vi "Auton Reaquire.vi"   [LabVIEW 2015]
uses:
  Robot Values.vi
types:
  T1 = typedef "Robot Values.ctl" = cluster{"Drive Motors":cluster{"Left Motor Value":dbl, "Right Motor Value":dbl, "Left Motor Encoder":dbl, "Right Motor Encoder":dbl, "High/Low Gear":bool}, "Sensors":cluster{"Gyro Angle":dbl, "Photoeye":bool, "Ultrasonic Range":dbl, "Shooter Speed Encoder":dbl, "Accelerometer Value":dbl, "Flashlight":bool, "Target Distance":dbl, "Target X Value":dbl, "Reset Gyro?":bool}, "Arms":cluster{"Desired Arm Position":dbl, "Left Arm Encoder":dbl, "Right Arm Encoder":dbl, "Left Arm Lower Limit":bool, "Right Arm Lower Limit":bool, "Initialize Arm Position?":bool}, "Acquisition and Scoring":cluster{"Acquiring?":bool, "Current Speed":dbl, "Setpoint Speed":dbl, "Prep Wheels":bool, "Shoot":bool, "Low Eject":bool, "Reverse Shooter Wheel":bool}, "Hanging":cluster{"Pivot Arms":dbl, "PTO":bool, "Left Pivot Encoder":dbl, "Right Pivot Encoder":dbl, "Hanging Pin":bool}}
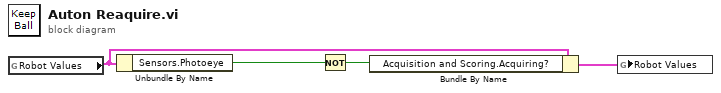
[diagram p0: block diagram]
diagram:
  n1 = global read "Robot Values.vi" "Robot Values"() -> (w4:T1)
  n2 = Unbundle By Name(w4) -> ("Sensors.Photoeye"=w3:bool)
  n3 = Not(x=w3) -> (.not. x?=w2:bool)
  n4 = Bundle By Name(cluster=w4, "Acquisition and Scoring.Acquiring?"=w2) -> (w1:T1)
  n5 = global write "Robot Values.vi" "Robot Values"(w1) -> ()
